vi "filePath.vi"() -> ()   [LabVIEW 2021]
panel:
  in  "Tdms_path":path
  in  "Path":path
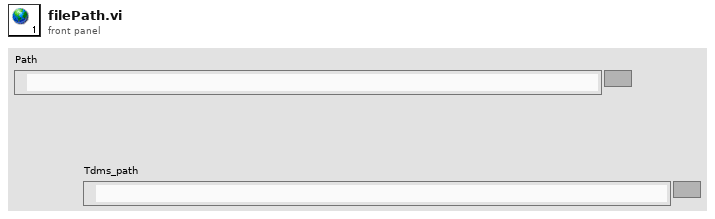
[diagram p1: front panel]
diagram:
